vi "Mark Field as Non-Default.vi"(0 "ZXing Options in":refnum<class "ZXing Options.lvclass">, 1 "Field":T1) -> (2 "ZXing Options out":refnum<class "ZXing Options.lvclass">)   [LabVIEW 2020, in "feature_detection.lvlib" / "ZXing Options.lvclass"]
uses:
  ZXing Options.lvclass
  Field.ctl
  ZXing Options.lvclass/ZXing Options.ctl
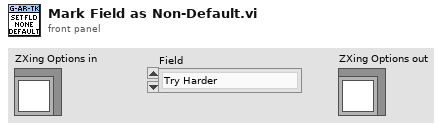
[diagram p1: front panel]
types:
  T1 = typedef "feature_detection.lvlib/ZXing Options.lvclass/Field.ctl" = enum8{"Try Harder", "Try Rotate", "Try Invert", "Try Downscale", "Is Pure", "Try Code 39 Ext Mode", "Return Errors", "Downscale Factor", "Min Line Count", "Max Number of Symbols", "Binarizer", "EAN Add On Symbol", "Text Mode", "Character Set", "Downscale Threshold"}
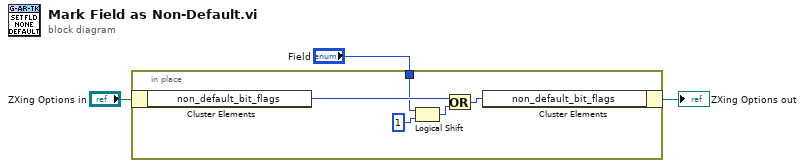
[diagram p0: block diagram]
diagram:
  n1 = in-place {
    in-place-border: "Field" -> [w4]
    n2 = in-place-cluster #1("ZXing Options in") -> ("non_default_bit_flags"=w6:u16)
    n3 = Logical Shift(y=w4, x=u16 1) -> (x << y=w7:u16)
    n4 = Or(x=w6, y=w7) -> (x .or. y?=w5:u16)
    n5 = in-place-cluster #1("non_default_bit_flags"=w5) -> (→"ZXing Options out":refnum<class "ZXing Options.lvclass">)
  }
